vi "Z calculator.vi"(9 "Blue":u16, 10 "Green":u16, 11 "Red":u16) -> (3 "Z":dbl)   [LabVIEW 2014, in "AMS TS3472 Light Sensor.lvlib" / "AMS TCS3472.lvclass"]
uses:
  AMS TCS3472.lvclass
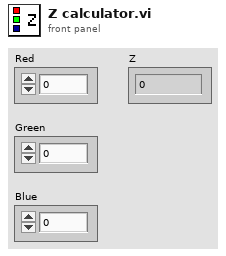
[diagram p1: front panel]
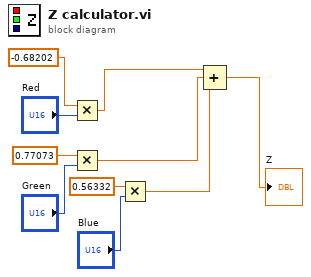
[diagram p0: block diagram]
diagram:
  n1 = Multiply(x=-0.68202, y="Red") -> (x*y=w4:dbl)
  n2 = Multiply(x=0.77073, y="Green") -> (x*y=w3:dbl)
  n3 = Multiply(x=0.56332, y="Blue") -> (x*y=w2:dbl)
  n4 = Compound Arithmetic op=ADD(w4, w3, w2) -> (→"Z":dbl)
